vi "Radau5_Get Vector U.vi"(0 "Delta In":dbl[](array[numeric]), 1 "Flag":bool, 5 "Stage time":dbl[](array[numeric]), 7 "Step Value Y":dbl[](array[numeric]), 9 "Vector Z in":dbl[](array[numeric]), 11 "Vector U in":dbl[](array[numeric]), 12 "Step size":dbl, 13 "Width":i32) -> (4 "Vector U Ready?":bool, 6 "Stage time out":dbl, 8 "Stage Y out":dbl[](array[numeric]), 10 "Stage Y' out":dbl[](array[numeric]), 15 "Vector U out":dbl[](array[numeric]))   [LabVIEW 2017, in "NI_DAE.lvlib"]
uses:
  <vilib>/gmath/NI_DAE.lvlib
  <vilib>/Analysis/Matrix/Datatypes/RealMatrix.ctl
  <vilib>/gmath/dae.llb/Radau5_Callback Status.ctl
  <vilib>/Analysis/7linalg.llb/Real Kronecker Product.vi
  <vilib>/Analysis/baseanly.llb/A x Vector (Optimized).vi
  <vilib>/Analysis/Matrix/Numeric/Multiply/Multiply - RM,R.vi
  <vilib>/Analysis/7linalg.llb/Create Special Real Matrix.vi
  <vilib>/Analysis/Matrix/NI_Matrix.lvlib
  <vilib>/Analysis/NI_AALPro.lvlib
  <vilib>/Analysis/NI_AALBase.lvlib
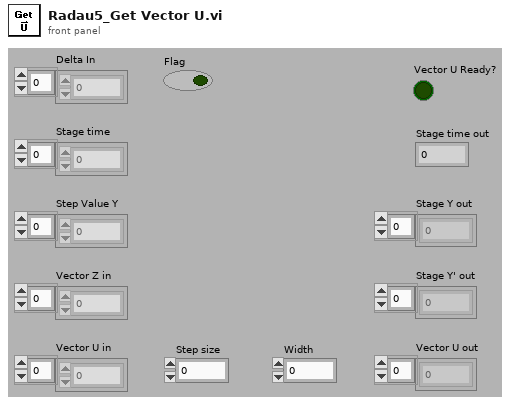
[diagram p1: front panel]
types:
  T1 = typedef "NI_Matrix.lvlib/RealMatrix.ctl" = dbl[][]
  T2 = typedef "NI_DAE.lvlib/Radau5_Callback Status.ctl" = enum16{"Before callback", "After callback"}
  T3 = enum32{"Identity", "Diagonal", "Toepliz", "Vandermonde", "Companion"}
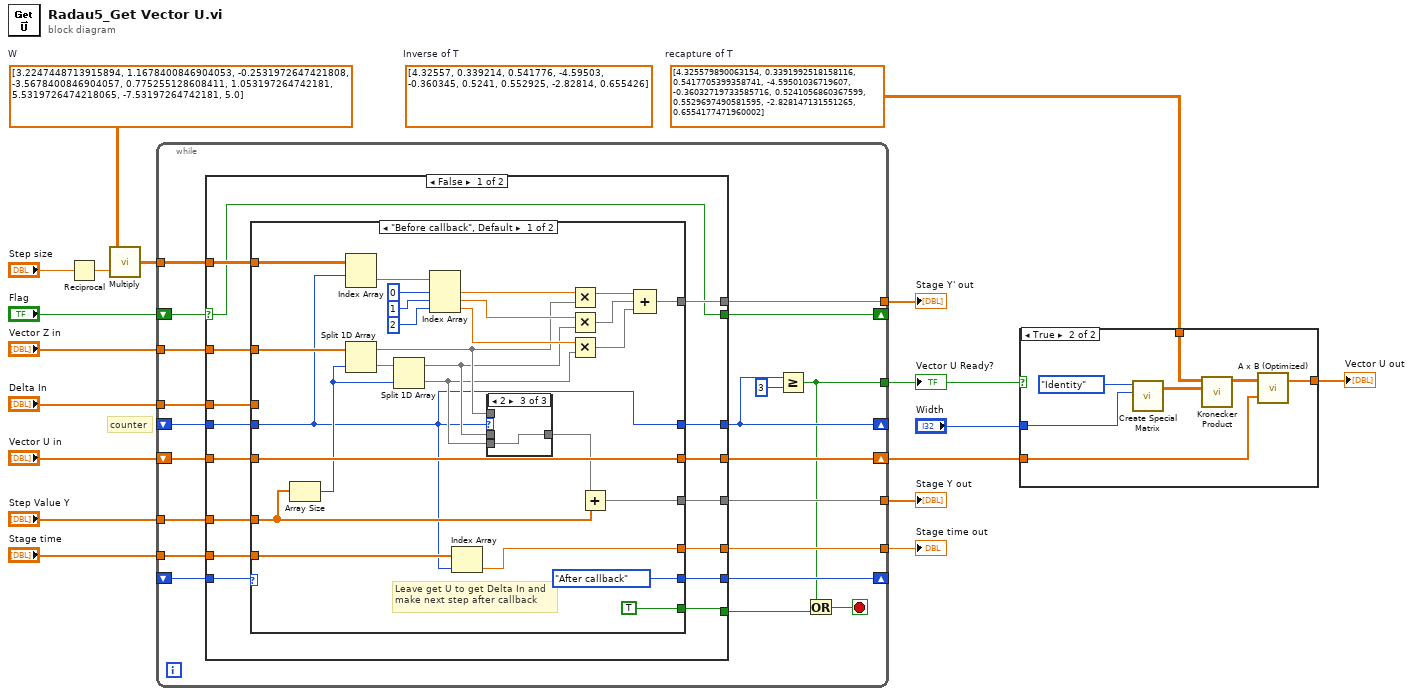
[diagram p0: block diagram]
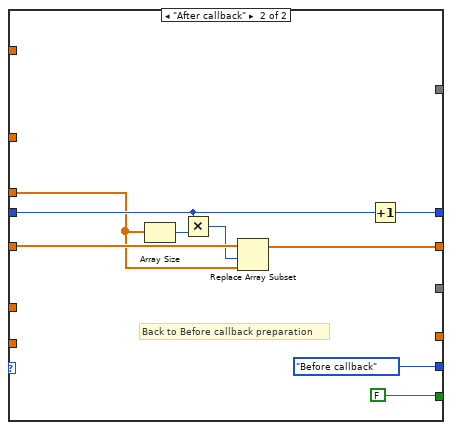
[diagram p5: hidden frame]
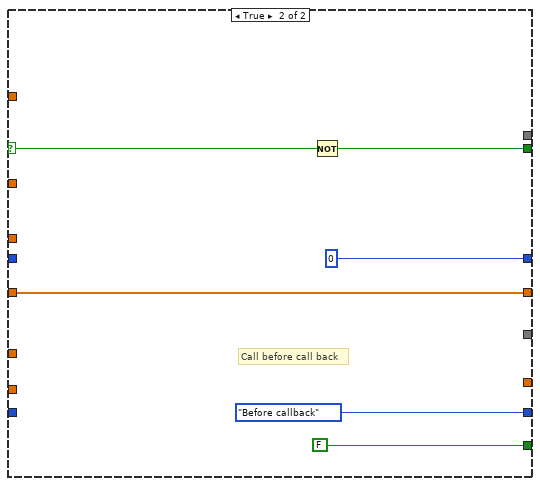
[diagram p6: hidden frame]
diagram:
  w1 = T1 [[4.325579890063154, 0.3391992518158116, 0.5417705399358741], [-4.59501036719607, -0.36032719733585716, 0.5241056860367599], [0.5529697490581595, -2.828147131551265, 0.6554177471960002]]  # recapture of T
  (unwired) T1 [[4.32557, 0.339214, 0.541776], [-4.59503, -0.360345, 0.5241], [0.552925, -2.82814, 0.655426]]  # Inverse of T
  w3 = T1 [[3.2247448713915894, 1.1678400846904053, -0.2531972647421808], [-3.5678400846904057, 0.775255128608411, 1.053197264742181], [5.5319726474218065, -7.53197264742181, 5.0]]  # W
  # "counter"
  n1 = Reciprocal(x="Step size") -> (1/x=w4:dbl)
  n2 = call-poly <vilib>:"Multiply.vi"("Real Scalar c"=w4, "Real Matrix A"=w3) -> ("A * c"=w2:T1)
  n3 = while {
    shift-right: [w38] -> _
    shift-left: _ -> [w36]
    tunnel: "Vector Z in" -> [w35]
    shift-right: [w23] -> _
    shift-left: _ -> [w34]
    tunnel: "Step Value Y" -> [w33]
    tunnel: [w32] -> w15
    tunnel: w2 -> [w31]
    tunnel: [w30] -> w9
    tunnel: "Stage time" -> [w29]
    tunnel: [w28] -> w12
    tunnel: "Delta In" -> [w27]
    shift-right: [w25] -> w7
    shift-left: "Vector U in" -> [w26]
    shift-right: [w24] -> _
    shift-left: "Flag" -> [w37]
    tunnel: [w20] -> w8
    stop <- w19 stop-if-true
    n4 = case shown="False" w37 {
      selector: w37 -> [w39 w96]
      tunnel: [w53 Radau5_Callback_Status."Before callback" ("Callback status")] -> w38
      tunnel: w36 -> [w54 _]
      tunnel: w35 -> [w52 _]
      tunnel: [w44 0] -> w23
      tunnel: w34 -> [w51 _]
      tunnel: w33 -> [w50 _]
      tunnel: [w49 _] -> w32
      tunnel: w31 -> [w48 _]
      tunnel: [w47 _] -> w30
      tunnel: w29 -> [w46 _]
      tunnel: [w45 _] -> w28
      tunnel: w27 -> [w43 _]
      tunnel: w26 -> [w42 w94]
      tunnel: [w41 w94] -> w25
      tunnel: [w40 FALSE] -> w21
      tunnel: [w39 w95] -> w24
      frame False {
        n5 = case shown="\"Before callback\", Default" w54 {
          tunnel: [Radau5_Callback_Status."After callback" ("Callback status") Radau5_Callback_Status."Before callback" ("Callback status")] -> w53
          tunnel: w52 -> [w63 _]
          tunnel: w51 -> [w56 w88]
          tunnel: w50 -> [w80 _]
          tunnel: [w79 _] -> w49
          tunnel: w48 -> [w78 _]
          tunnel: [w55 _] -> w47
          tunnel: w46 -> [w67 _]
          tunnel: [w66 _] -> w45
          tunnel: [w56 w93] -> w44
          tunnel: w43 -> [_ w85]
          tunnel: w42 -> [w65 w91]
          tunnel: [w65 w90] -> w41
          tunnel: [TRUE FALSE] -> w40
          frame "Before callback", Default {
            # "Leave get U to get Delta In and\nmake next step after callback"
            n6 = Array Size(array=w80) -> (size(s)=w61:i32)
            n7 = Index Array(array=w78, index (row)=w56) -> (element=w77:dbl[])  [unwired: 1 in]
            n8 = Split 1D Array(array=w63, index=w61) -> (first subarray=w60:dbl[], second subarray=w62:dbl[])
            n9 = Split 1D Array(array=w62, index=w61) -> (first subarray=w59:dbl[], second subarray=w58:dbl[])
            n10 = Index Array(array=w77, index #1=0 ("index"), index #2=1 ("index"), index #3=2 ("index")) -> (element #1=w73:dbl, element #2=w72:dbl, element #3=w71:dbl)
            n11 = Index Array(array=w67, index=w56) -> (element=w66:dbl)
            n12 = case shown="2" w56 {
              tunnel: w60 -> [w82 _ _]
              tunnel: w59 -> [_ w83 _]
              tunnel: w58 -> [_ _ w84]
              tunnel: [w82 w83 w84] -> w57
              frame 0, Default {
              }
              frame 1 {
              }
              frame 2 {
              }
            }
            n13 = Multiply(x=w73, y=w60) -> (x*y=w70:dbl[])
            n14 = Multiply(x=w72, y=w59) -> (x*y=w69:dbl[])
            n15 = Multiply(x=w71, y=w58) -> (x*y=w68:dbl[])
            n16 = Add(x=w57, y=w80) -> (x+y=w79:dbl[])
            n17 = Compound Arithmetic op=ADD(w70, w69, w68) -> (w55:dbl[])
          }
          frame "After callback" {
            # "Back to Before callback preparation"
            n18 = Array Size(array=w85) -> (size(s)=w87:i32)
            n19 = Multiply(x=w88, y=w87) -> (x*y=w86:i32)
            n20 = Replace Array Subset(array=w91, new element=w85, index=w86) -> (w90:dbl[])
            n21 = Increment(x=w88) -> (x+1=w93:i32)
          }
        }
      }
      frame True {
        # "Call before call back"
        n22 = Not(x=w96) -> (.not. x?=w95:bool)
      }
    }
    n23 = Greater Or Equal?(x=w23, y=3) -> (x >= y?=w20:bool)
    n24 = Or(x=w20, y=w21) -> (x .or. y?=w19:bool)
  }
  "Vector U Ready?" <- w8
  "Stage time out" <- w12
  "Stage Y out" <- w15
  "Stage Y' out" <- w9
  n25 = case shown="True" w8 {
    tunnel: w1 -> [_ w107]
    tunnel: w7 -> [w100 w105]
    tunnel: [w100 w104] -> w6
    tunnel: "Width" -> [_ w103]
    frame False {
    }
    frame True {
      n26 = call-poly <vilib>:"Create Special Matrix.vi"("matrix type"=T3."Identity", "matrix size"=w103) -> ("Special Matrix"=w102:T1)  [unwired: 3 in, 1 out]
      n27 = call-poly <vilib>:"Kronecker Product.vi"("B"=w102, "A"=w107) -> ("Kronecker Product"=w106:T1)  [unwired: 9 out]
      n28 = call-poly <vilib>:"A x B (Optimized).vi"("Vector"=w105, "A"=w106) -> ("A x Vector"=w104:dbl[])  [unwired: 1 out]
    }
  }
  "Vector U out" <- w6
